vi "set Removable.vi"(8 "error in (no error)":errorcluster, 10 "Removable":bool, 11 "xceDataNode in":refnum<class "xceDataNode.lvclass">) -> (0 "error out":errorcluster, 3 "xceDataNode out":refnum<class "xceDataNode.lvclass">)   [LabVIEW 2013, in "xceDataNode.lvclass"]
doc: "Set Removable. Determines if a node can be removed from the tree data structure."
uses:
  xceDataNode.lvclass
  xceDataNode.lvclass/xceDataNode.ctl
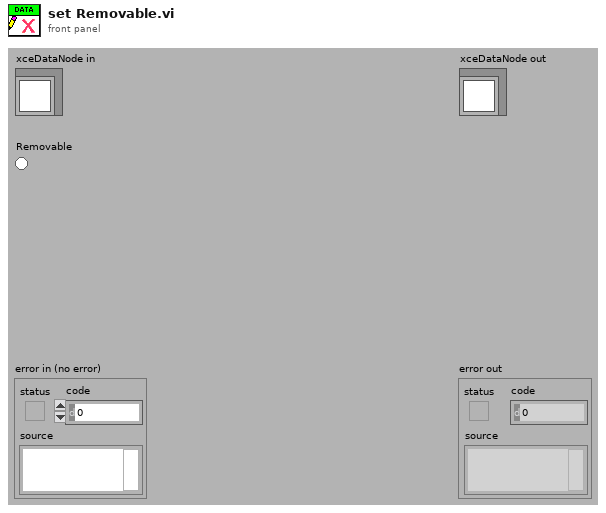
[diagram p1: front panel]
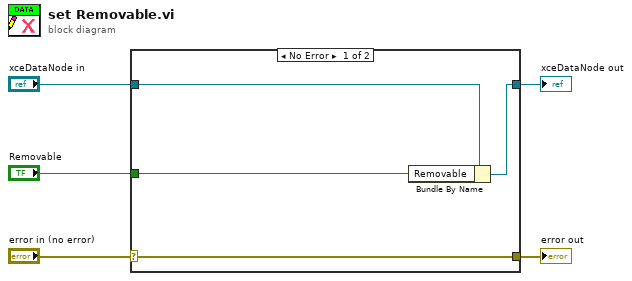
[diagram p0: block diagram]
diagram:
  n1 = case shown="No Error" "error in (no error)" {
    selector: "error in (no error)" -> [w9 w10]
    tunnel: [w9 w10] -> w4
    tunnel: [w7 w11] -> w2
    tunnel: "xceDataNode in" -> [w8 w11]
    tunnel: "Removable" -> [w6 _]
    frame No Error {
      n2 = Bundle By Name(cluster=w8, "Removable"=w6) -> (w7:refnum<class "xceDataNode.lvclass">)
    }
    frame Error {
    }
  }
  "error out" <- w4
  "xceDataNode out" <- w2
